vi "Open Stimulator_cluster v2.vi"(7 "Stimulator":T1={"Log File In"=refnum, "Stimulator In"="", "Stimulator Mode"="", "Log Data"=FALSE, "Doublet/Triplet  Interval"=0.0, "Stim Frequency"=0.0, "N-Factor"=0, "Active Channels"=[], "Low-Frequency Channels"=[], "Stimulator State"=enum."Closed", "Mode Array"=[], "Current Array"=[], "Pulse Duration Array"=[], "VISA Timeout"=50}) -> (1 "Log Entry":string, 2 "Stim Open":bool caption="Stim Open?", 3 "Stimulator":T1={"Log File In"=refnum, "Stimulator In"="", "Stimulator Mode"="", "Log Data"=FALSE, "Doublet/Triplet  Interval"=0.0, "Stim Frequency"=0.0, "N-Factor"=0, "Active Channels"=[], "Low-Frequency Channels"=[], "Stimulator State"=enum."Closed", "Mode Array"=[], "Current Array"=[], "Pulse Duration Array"=[], "VISA Timeout"=50})   [LabVIEW 2019]
uses:
  Controls/Stimulator Cluster.ctl
  Controls/Stimulator Mode.ctl
  Version 2/Data Type Defs/Pulse Mode (array).ctl
  Controls/Stim Current Array.ctl
  Controls/Pulse Duration Array.ctl
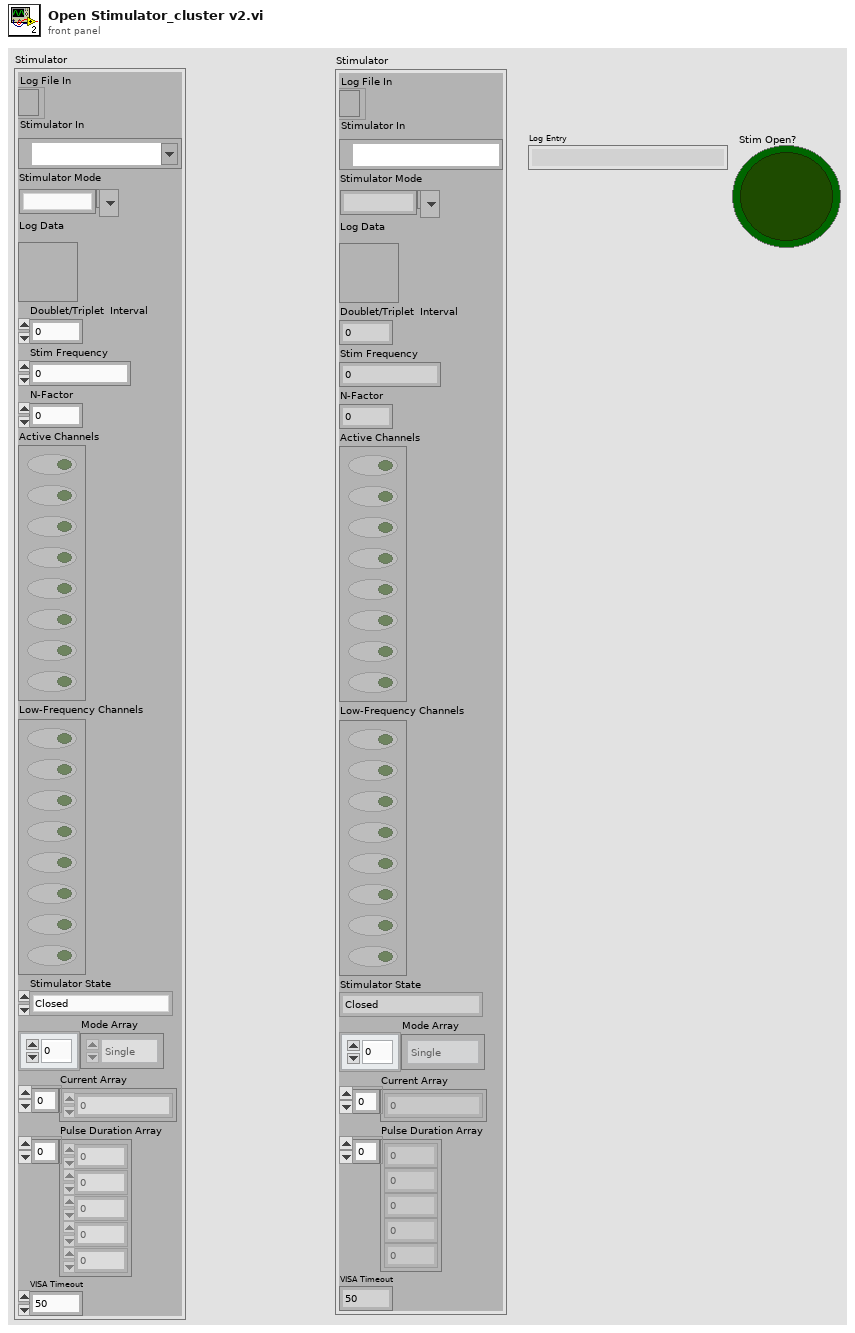
[diagram p1: front panel]
types:
  T1 = typedef "Stimulator Cluster.ctl" = cluster{"Log File In":refnum<file>, "Stimulator In":refnum<visa-resource-name>, "Stimulator Mode":T2, "Log Data":bool, "Doublet/Triplet  Interval":dbl, "Stim Frequency":dbl, "N-Factor":u8, "Active Channels":bool[], "Low-Frequency Channels":bool[], "Stimulator State":enum16{"Closed", "Open", "Initialized", "Stimulating"}, "Mode Array":T3, "Current Array":T4, "Pulse Duration Array":T5, "VISA Timeout":u32}
  T2 = typedef "Stimulator Mode.ctl" = string
  T3 = typedef "Pulse Mode (array).ctl" = enum16{"Single", "Doublet", "Triplet"}[]
  T4 = typedef "Stim Current Array.ctl" = u8[]
  T5 = typedef "Pulse Duration Array.ctl" = u32[]
  T6 = cluster{"Command Name":string, "Command String":string, "Log String":string, "Response":string, "Stimulator":string}
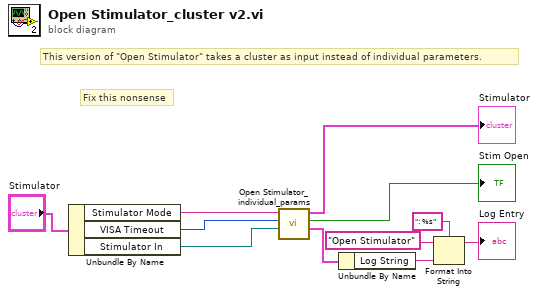
[diagram p0: block diagram]
diagram:
  # "Fix this nonsense"
  # "This version of \"Open Stimulator\" takes a cluster as input instead of individual parameters."
  n1 = Unbundle By Name("Stimulator") -> ("Stimulator Mode"=w3:T2, "VISA Timeout"=w2:u32, "Stimulator In"=w1:refnum<visa-resource-name>)
  n2 = call "Open Stimulator_individual_params.vi"("Stimulator Name"=w1, "timeout (ms)"=w2, "Stimulator Mode"=w3) -> ("Open Stim Result"=w11:T6, "Stim Open"=→"Stim Open":bool, "Stimulator"=→"Stimulator":T1)  [unwired: 1 in, 1 out]
  n3 = Unbundle By Name(w11) -> ("Log String"=w10:string)
  n4 = Format Into String(format string=": %s", initial string="Open Stimulator", w10) -> (resulting string=→"Log Entry":string)  [unwired: 1 in, 1 out]
